vi "Create Conpane Map.vi"(8 "error in":errorcluster, 9 "Ref.Name VI (Interface)":refnum<vi>, 10 "Control FP Order":i32[](array[numeric])) -> (0 "error out":errorcluster, 2 "Conpane Map":T1(c390))   [LabVIEW 2025, in "_Msg Rescript.lvlib" / "_Msg Rescript.lvclass"]
uses:
  _Msg Rescript.lvclass
  _Msg Rescript.lvclass/_Msg Rescript.ctl
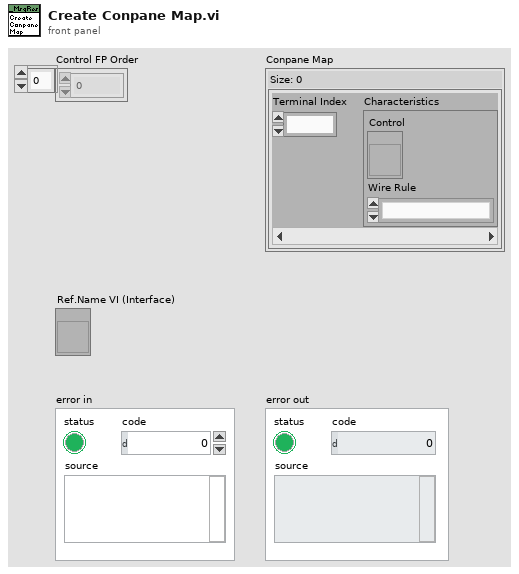
[diagram p1: front panel]
types:
  T1 = map{i32, cluster{"Control":refnum<vi>, "Wire Rule":enum16{"Invalid Wire Rule", "Required", "Recommended", "Optional", "Dynamic Dispatch"}}}
  T2 = enum16{"Invalid Wire Rule", "Required", "Recommended", "Optional", "Dynamic Dispatch"}[]
  T3 = cluster{"Control":refnum<vi>, "Wire Rule":enum16{"Invalid Wire Rule", "Required", "Recommended", "Optional", "Dynamic Dispatch"}}
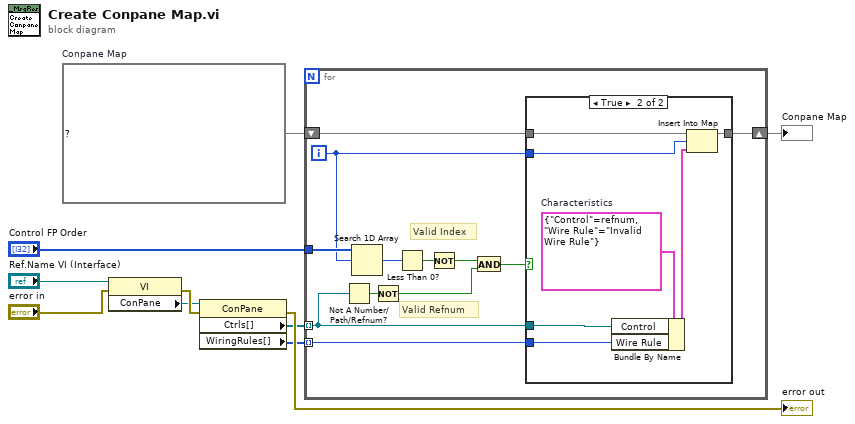
[diagram p0: block diagram]
diagram:
  w7 = T1 {}  # Conpane Map
  n1 = property class="VI"(reference="Ref.Name VI (Interface)", error in="error in") -> (error out=w9:errorcluster, "ConPane"=w8:refnum<vi>)  [unwired: 1 out]
  n2 = property class="ConPane"(reference=w8, error in=w9) -> (error out=→"error out":errorcluster, "Ctrls[]"=w1:refnum<vi>[], "WiringRules[]"=w6:T2)  [unwired: 1 out]
  n3 = for {
    tunnel: "Control FP Order" -> [w19]
    shift-right: [w22] -> w3
    shift-left: w7 -> [w21]
    tunnel: w1 -> [w17] mode=indexing
    tunnel: w6 -> [w20] mode=indexing
    i -> [w18]
    # "Valid Refnum"
    # "Valid Index"
    n4 = Not A Number/Path/Refnum?(number/path/refnum=w17) -> (NaN/Path/Refnum?=w16:bool)
    n5 = Search 1D Array(1D array=w19, element=w18) -> (index of element=w13:i32)  [unwired: 1 in]
    n6 = Not(x=w16) -> (.not. x?=w15:bool)
    n7 = Less Than 0?(x=w13) -> (x < 0?=w12:bool)
    n8 = Not(x=w12) -> (.not. x?=w11:bool)
    n9 = And(x=w11, y=w15) -> (x .and. y?=w14:bool)
    n10 = case shown="True" w14 {
      tunnel: [w23 w30] -> w22
      tunnel: w21 -> [w23 w29]
      tunnel: w20 -> [_ w28]
      tunnel: w18 -> [_ w27]
      tunnel: w17 -> [_ w26]
      frame False {
      }
      frame True {
        w25 = T3 {"Control"=refnum, "Wire Rule"=enum."Invalid Wire Rule"}  # Characteristics
        n11 = Bundle By Name(cluster=w25, "Control"=w26, "Wire Rule"=w28) -> (w24:T3)
        n12 = Insert Into Map(map in=w29, key=w27, value=w24) -> (map out=w30:T1)  [unwired: 2 out]
      }
    }
  }
  "Conpane Map" <- w3
